vi "ITR HP BAE3.vi"(5 "input":dbl format="%.2f", 7 "T (corner period) [steps]":dbl(slide)=10.237739663395852 scale=1.0..1000.0) -> (8 "output":dbl format="%.2f")   [LabVIEW 2014]
doc: "ITR High Pass Filter\nCalculates recursively to create a high pass filter.\n\nVi(j) = current input voltage\nVo(j) = current output voltage\nVi(j-1) = previous input voltage\nVo(j-1) = previous output voltage\nT = corner period / decay constant [number of time steps]\nb = relates to corner period [per number of time steps]\n \nb = 2* pi / T \nVo(j) = [Vo(j-1)+Vi(j)-Vi(j-1)]/[b+1]\n\nBeverly Abadines\nPHY 350: E3"
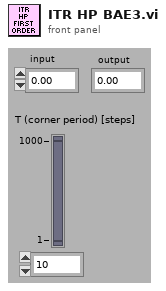
[diagram p1: front panel]
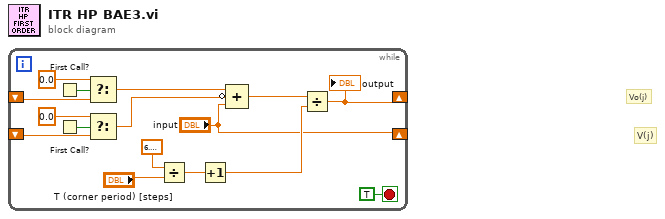
[diagram p0: block diagram]
diagram:
  # "V(j)"
  # "Vo(j)"
  n1 = while {
    shift-left: _ -> [w2]
    shift-right: [w10] -> _
    shift-right: ["input"] -> _
    shift-left: _ -> [w5]
    stop <- TRUE stop-if-true
    n2 = First Call?() -> (First Call?: T/F=w4:bool)
    n3 = First Call?() -> (First Call?: T/F=w9:bool)
    n4 = Select(t=0.0, s=w4, f=w2) -> (s? t:f=w1:dbl)
    n5 = Select(t=0.0, s=w9, f=w5) -> (s? t:f=w7:dbl)
    n6 = Divide(x=6.283185307179586, y="T (corner period) [steps]") -> (x/y=w14:dbl)
    n7 = Increment(x=w14) -> (x+1=w13:dbl)
    n8 = Compound Arithmetic op=ADD(w1, invert w7, "input") -> (w11:dbl)
    n9 = Divide(x=w11, y=w13) -> (x/y=w10:dbl)
    "output" <- w10
  }
